vi "MB Serial Master Query Write Multiple Registers (poly).vi"(0 "VISA resource name":refnum<visa-resource-name>, 1 "MB status in":T1 {"MB update(s)" format="%.2g"; "ProCoDA Request"."PC update (s)" format="%.2f"; "ProCoDA Request"."# registers" min=1}, 3 "MB ID-Address in":T4, 4 "Timeout":u32=500, 5 "error in":errorcluster) -> (14 "VISA resource name out":refnum<visa-resource-name>, 15 "MB status out":T1 {"MB update(s)" format="%.2g"; "ProCoDA Request"."PC update (s)" format="%.2f"; "ProCoDA Request"."# registers" min=1}, 16 "Exception Code":u8 format="%.0x", 19 "error out":errorcluster)   [LabVIEW 2019]
doc: "The master uses this VI to write multiple registers to the slave. This corresponds to a public function code of 16 in the MODBUS protocol."
uses:
  MB ID-Address.ctl
  SerialParameters.ctl
  MB status.ctl
  ProCoDA MB Request.ctl
  Read Write.ctl
  MB Modbus Command.ctl
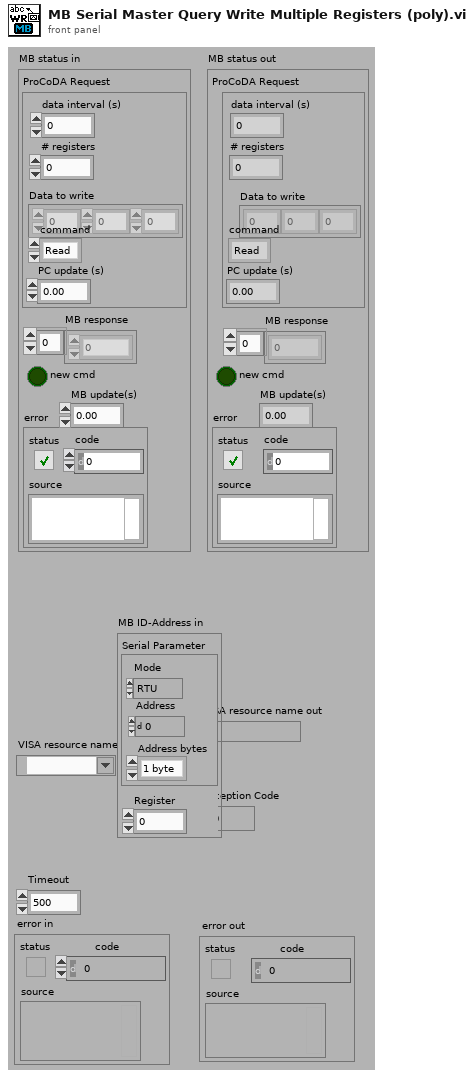
[diagram p1: front panel]
types:
  T1 = typedef "MB status.ctl" = cluster{"ProCoDA Request":T2, "MB response":dbl[], "new cmd":bool, "error":errorcluster, "MB update(s)":dbl}
  T2 = typedef "ProCoDA MB Request.ctl" = cluster{"# registers":u8, "Data to write":u16[], "data interval (s)":dbl, "command":T3, "PC update (s)":dbl}
  T3 = typedef "Read Write.ctl" = enum16{"Read", "Write"}
  T4 = typedef "MB ID-Address.ctl" = cluster{"Serial Parameter":T5, "Register":u16}
  T5 = typedef "SerialParameters.ctl" = cluster{"Mode":enum16{"RTU", "ASCII"}, "Address":u16, "Address bytes":enum16{"1 byte", "2 bytes"}}
  T6 = typedef "MB Modbus Command.ctl" = cluster{"Function Code":u8, "Starting Address":u16, "Quantity":u16, "Data":u16[], "Discrete":bool[]}
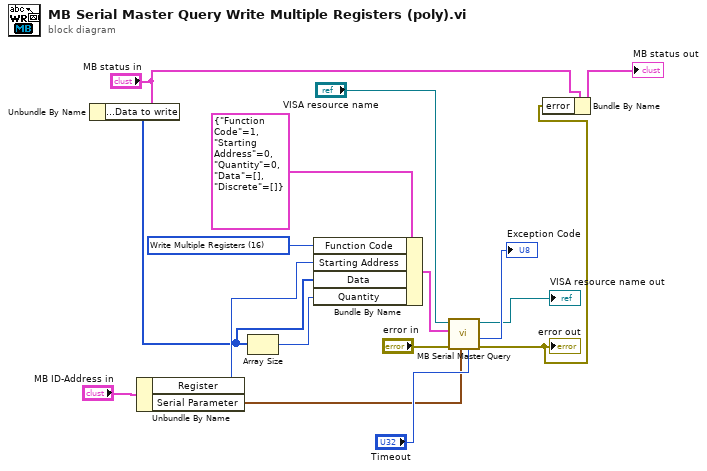
[diagram p0: block diagram]
diagram:
  w14 = u8 16 items=["Read Coils"=1, "Read Discrete Inputs"=2, "Read Holding Registers"=3, "Read Input Registers"=4, "Write Single Coil"=5, "Write Single Register"=6, "Read Exception Status"=7, "Write Multiple Coils"=15, "Write Multiple Registers"=16] ("Function Code")
  n1 = Unbundle By Name("MB status in") -> ("ProCoDA Request.Data to write"=w6:u16[])
  n2 = Unbundle By Name("MB ID-Address in") -> ("Register"=w7:u16, "Serial Parameter"=w1:T5)
  n3 = Array Size(array=w6) -> (size(s)=w9:i32)
  n4 = Bundle By Name(cluster=T6 {"Function Code"=1, "Starting Address"=0, "Quantity"=0, "Data"=[], "Discrete"=[]} ("Modbus Command"), "Function Code"=w14, "Starting Address"=w7, "Data"=w6, "Quantity"=w9) -> (w15:T6)
  n5 = call "MB Serial Master Query.vi"("Timeout"="Timeout", "Serial Parameters"=w1, "error in (no error)"="error in", "Modbus Command"=w15, "VISA resource name"="VISA resource name") -> ("error out"=w2:errorcluster, "Exception Code"=→"Exception Code":u8, "VISA resource name out"=→"VISA resource name out":refnum<visa-resource-name>)  [unwired: 2 in, 2 out]
  "error out" <- w2
  n6 = Bundle By Name(cluster="MB status in", "error"=w2) -> (→"MB status out":T1)
